vi "Assignment_01.vi"() -> ()   [LabVIEW 2020]
panel:
  out "Mixed Signal Graph":cluster{dbl[], dbl[], dbl[], dbl[]}(graph)
  out "h(n)":dbl[](array[numeric])
  out "Y (Zero Input)":dbl[](array[numeric])
  out "Y (Zero State)":dbl[](array[numeric])
  out "Y (Total)":dbl[](array[numeric])
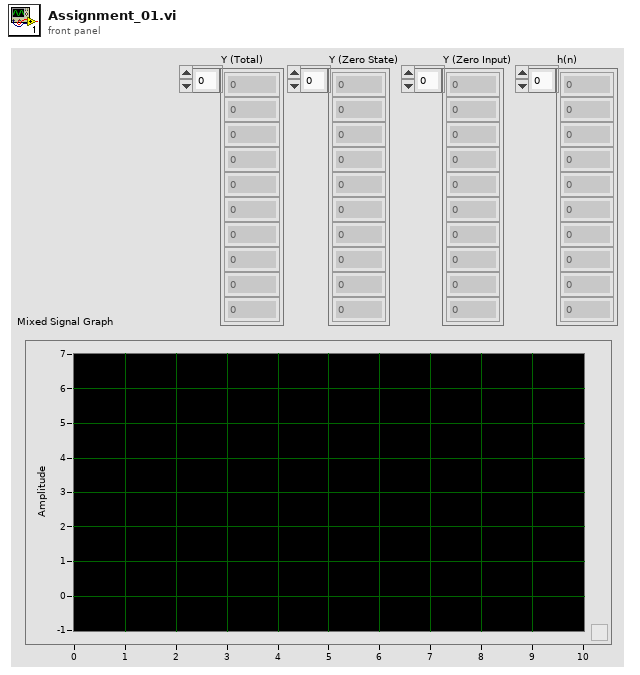
[diagram p1: front panel]
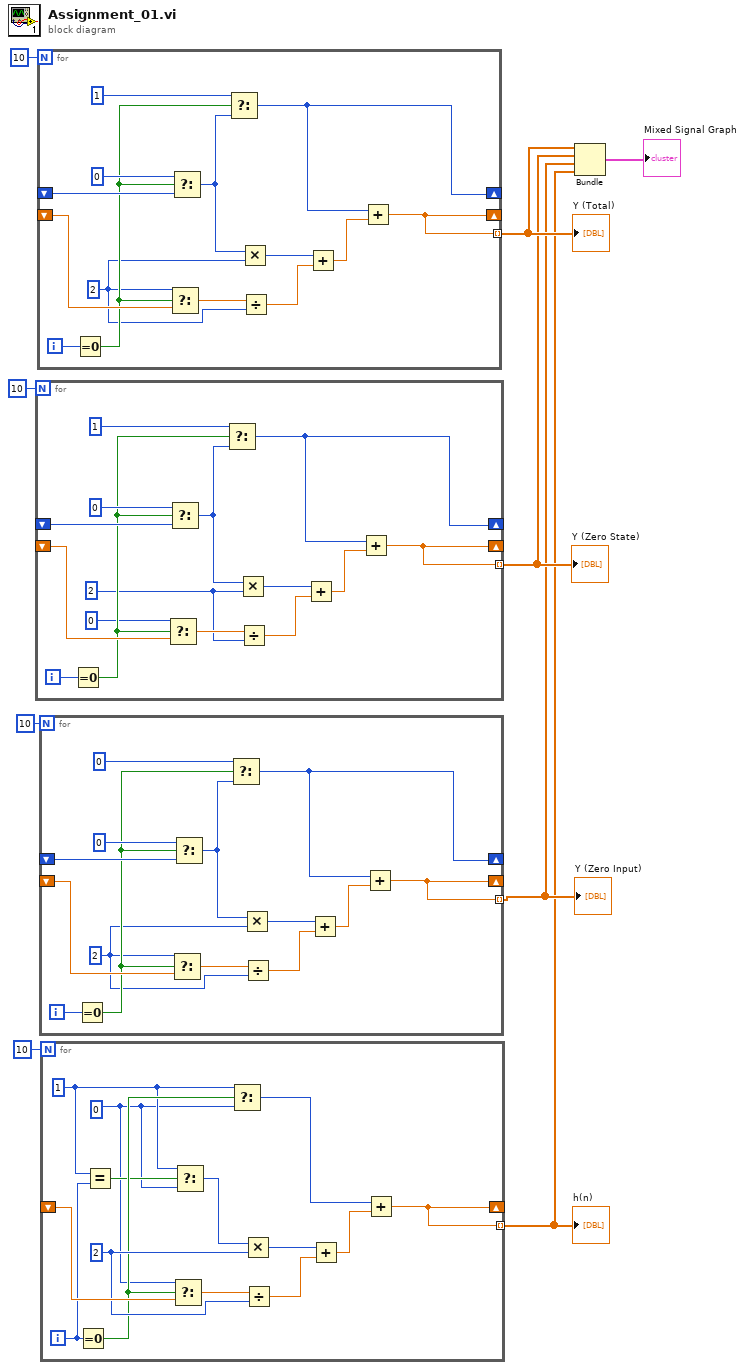
[diagram p0: block diagram]
diagram:
  n1 = for {
    N: 10 -> [_]
    shift-right: [w14] -> _
    shift-left: _ -> [w21]
    shift-right: [w12] -> _
    shift-left: _ -> [w24]
    tunnel: [w12] -> w6 mode=indexing
    i -> [w11]
    w10 = 2
    n2 = Equal To 0?(x=w11) -> (x = 0?=w20:bool)
    n3 = Select(t=0, s=w20, f=w24) -> (s? t:f=w23:dbl)
    n4 = Select(t=0, s=w20, f=w21) -> (s? t:f=w18:i32)
    n5 = Select(t=1, s=w20, f=w18) -> (s? t:f=w14:i32)
    n6 = Multiply(x=w18, y=w10) -> (x*y=w16:i32)
    n7 = Divide(x=w23, y=w10) -> (x/y=w15:dbl)
    n8 = Add(x=w16, y=w15) -> (x+y=w13:dbl)
    n9 = Add(x=w14, y=w13) -> (x+y=w12:dbl)
  }
  "Y (Zero State)" <- w6
  n10 = for {
    N: 10 -> [_]
    shift-right: [w28] -> _
    shift-left: _ -> [w35]
    shift-right: [w26] -> _
    shift-left: _ -> [w38]
    tunnel: [w26] -> w8 mode=indexing
    i -> [w25]
    w31 = 2
    n11 = Equal To 0?(x=w25) -> (x = 0?=w34:bool)
    n12 = Select(t=w31, s=w34, f=w38) -> (s? t:f=w37:dbl)
    n13 = Select(t=0, s=w34, f=w35) -> (s? t:f=w32:i32)
    n14 = Select(t=1, s=w34, f=w32) -> (s? t:f=w28:i32)
    n15 = Multiply(x=w32, y=w31) -> (x*y=w30:i32)
    n16 = Divide(x=w37, y=w31) -> (x/y=w29:dbl)
    n17 = Add(x=w30, y=w29) -> (x+y=w27:dbl)
    n18 = Add(x=w28, y=w27) -> (x+y=w26:dbl)
  }
  "Y (Total)" <- w8
  n19 = for {
    N: 10 -> [_]
    shift-right: [w42] -> _
    shift-left: _ -> [w49]
    shift-right: [w40] -> _
    shift-left: _ -> [w52]
    tunnel: [w40] -> w3 mode=indexing
    i -> [w39]
    w45 = 2
    n20 = Equal To 0?(x=w39) -> (x = 0?=w48:bool)
    n21 = Select(t=w45, s=w48, f=w52) -> (s? t:f=w51:dbl)
    n22 = Select(t=0, s=w48, f=w49) -> (s? t:f=w46:i32)
    n23 = Select(t=0, s=w48, f=w46) -> (s? t:f=w42:i32)
    n24 = Multiply(x=w46, y=w45) -> (x*y=w44:i32)
    n25 = Divide(x=w51, y=w45) -> (x/y=w43:dbl)
    n26 = Add(x=w44, y=w43) -> (x+y=w41:dbl)
    n27 = Add(x=w42, y=w41) -> (x+y=w40:dbl)
  }
  "Y (Zero Input)" <- w3
  n28 = for {
    N: 10 -> [_]
    shift-right: [w59] -> _
    shift-left: _ -> [w66]
    tunnel: [w59] -> w1 mode=indexing
    i -> [w56]
    w53 = 0
    w54 = 1
    w64 = 2
    n29 = Equal To 0?(x=w56) -> (x = 0?=w57:bool)
    n30 = Equal?(x=w54, y=w56) -> (x = y?=w55:bool)
    n31 = Select(t=w53, s=w57, f=w66) -> (s? t:f=w65:dbl)
    n32 = Select(t=w54, s=w55, f=w53) -> (s? t:f=w58:i32)
    n33 = Select(t=w54, s=w57, f=w53) -> (s? t:f=w61:i32)
    n34 = Multiply(x=w58, y=w64) -> (x*y=w63:i32)
    n35 = Divide(x=w65, y=w64) -> (x/y=w62:dbl)
    n36 = Add(x=w63, y=w62) -> (x+y=w60:dbl)
    n37 = Add(x=w61, y=w60) -> (x+y=w59:dbl)
  }
  "h(n)" <- w1
  n38 = Bundle(w8, w6, w3, w1) -> (→"Mixed Signal Graph":cluster{dbl[], dbl[], dbl[], dbl[]})  [unwired: 1 in]
